vi "Array2MergedSignal.vi"(10 "Array":dbl[](array[numeric])) -> (0 "Dynamic Data Type 6":dbl, 1 "Dynamic Data Type 5":dbl, 2 "Dynamic Data Type 4":dbl, 3 "Dynamic Data Type 3":dbl, 4 "Dynamic Data Type 7":dbl, 5 "Dynamic Data Type 2":dbl, 6 "Dynamic Data Type 8":dbl, 7 "Dynamic Data Type":dbl, 8 "Dynamic Data Type 10":dbl, 11 "Dynamic Data Type 9":dbl)   [LabVIEW 2023]
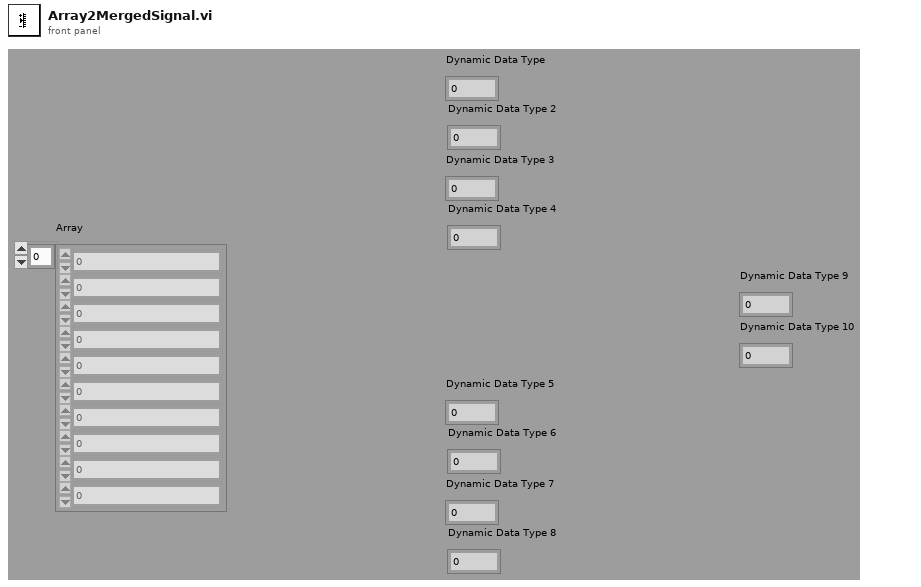
[diagram p1: front panel]
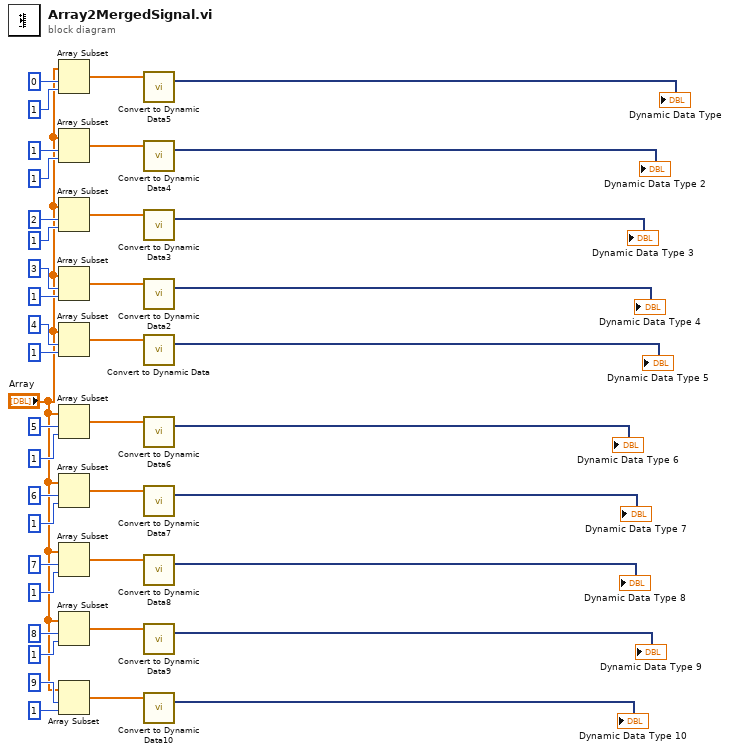
[diagram p0: block diagram]
diagram:
  n1 = Array Subset "Array Subset"(array="Array", index=0, length=1) -> (w12:dbl[])
  n2 = Array Subset "Array Subset"(array="Array", index=1, length=1) -> (w14:dbl[])
  n3 = Array Subset "Array Subset"(array="Array", index=2, length=1) -> (w16:dbl[])
  n4 = Array Subset "Array Subset"(array="Array", index=3, length=1) -> (w18:dbl[])
  n5 = Array Subset "Array Subset"(array="Array", index=4, length=1) -> (w20:dbl[])
  n6 = Array Subset "Array Subset"(array="Array", index=5, length=1) -> (w10:dbl[])
  n7 = Array Subset "Array Subset"(array="Array", index=6, length=1) -> (w8:dbl[])
  n8 = Array Subset "Array Subset"(array="Array", index=7, length=1) -> (w6:dbl[])
  n9 = Array Subset "Array Subset"(array="Array", index=8, length=1) -> (w4:dbl[])
  n10 = Array Subset "Array Subset"(array="Array", index=9, length=1) -> (w2:dbl[])
  n11 = call "Convert to Dynamic Data5"("Array"=w12) -> ("Dynamic Data Type"=→"Dynamic Data Type":dynamicdata)  [unwired: 3 in]
  n12 = call "Convert to Dynamic Data4"("Array"=w14) -> ("Dynamic Data Type"=→"Dynamic Data Type 2":dynamicdata)  [unwired: 3 in]
  n13 = call "Convert to Dynamic Data3"("Array"=w16) -> ("Dynamic Data Type"=→"Dynamic Data Type 3":dynamicdata)  [unwired: 3 in]
  n14 = call "Convert to Dynamic Data2"("Array"=w18) -> ("Dynamic Data Type"=→"Dynamic Data Type 4":dynamicdata)  [unwired: 3 in]
  n15 = call "Convert to Dynamic Data"("Array"=w20) -> ("Dynamic Data Type"=→"Dynamic Data Type 5":dynamicdata)  [unwired: 3 in]
  n16 = call "Convert to Dynamic Data6"("Array"=w10) -> ("Dynamic Data Type"=→"Dynamic Data Type 6":dynamicdata)  [unwired: 3 in]
  n17 = call "Convert to Dynamic Data7"("Array"=w8) -> ("Dynamic Data Type"=→"Dynamic Data Type 7":dynamicdata)  [unwired: 3 in]
  n18 = call "Convert to Dynamic Data8"("Array"=w6) -> ("Dynamic Data Type"=→"Dynamic Data Type 8":dynamicdata)  [unwired: 3 in]
  n19 = call "Convert to Dynamic Data9"("Array"=w4) -> ("Dynamic Data Type"=→"Dynamic Data Type 9":dynamicdata)  [unwired: 3 in]
  n20 = call "Convert to Dynamic Data10"("Array"=w2) -> ("Dynamic Data Type"=→"Dynamic Data Type 10":dynamicdata)  [unwired: 3 in]
